vi "RGB to HSL.vi"(8 "Error In":errorcluster, 9 "Blue":u8, 10 "Green":u8, 11 "Red":u8) -> (0 "Error Out":errorcluster, 1 "Lum":u8, 2 "Sat":u8, 3 "Hue":u8)   [LabVIEW 2012, in "Picture Box Tools.lvlib"]
doc: "Converts RGB values (0-255) to HSL values (0-240). RGB colorspace is the display colorspace for web and computer monitors. RGB uses Red, Green and Blue components to form a color. This isn't very useful for programmatically changing a color. HSL colorspace uses Hue, Saturation and Lightness components of a color which can be analyzed, extract or modified in a way to change the function of a color. \n\nSee HSLToolsBasicExample.vi for more information in the NI Example Finder."
uses:
  Picture Box Tools.lvlib
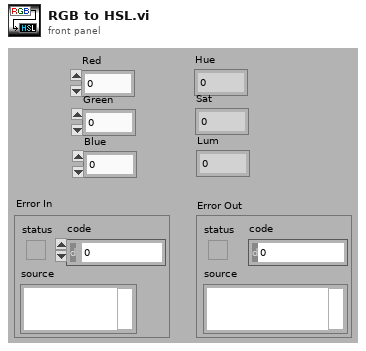
[diagram p1: front panel]
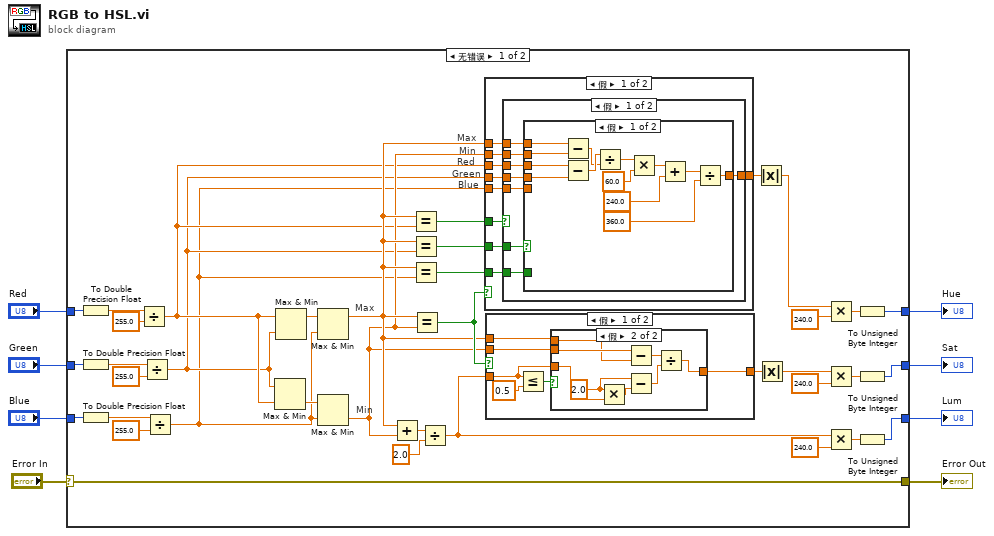
[diagram p0: block diagram]
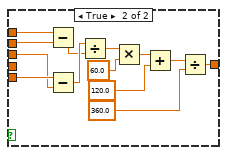
[diagram p2: hidden frame]
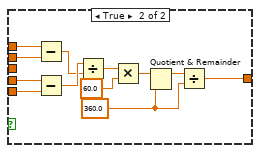
[diagram p3: hidden frame]
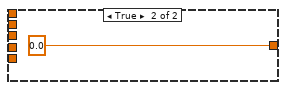
[diagram p4: hidden frame]
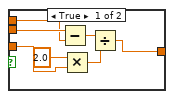
[diagram p5: hidden frame]
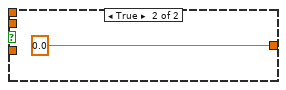
[diagram p6: hidden frame]
diagram:
  n1 = case shown="无错误" "Error In" {
    selector: "Error In" -> [w21 w124]
    tunnel: [w9 w127] -> w8
    tunnel: "Red" -> [w20 w127]
    tunnel: "Green" -> [w19 w126]
    tunnel: "Blue" -> [w18 w125]
    tunnel: [w10 w126] -> w4
    tunnel: [w11 w125] -> w3
    tunnel: [w21 w124] -> w1
    frame No Error {
      # "Blue"
      # "Green"
      # "Red"
      # "Min"
      # "Max"
      # "Min"
      # "Max"
      n2 = To Double Precision Float(number=w20) -> (double precision float=w17:dbl)
      n3 = To Double Precision Float(number=w19) -> (double precision float=w16:dbl)
      n4 = To Double Precision Float(number=w18) -> (double precision float=w15:dbl)
      n5 = Divide(x=w17, y=255.0) -> (x/y=w26:dbl)
      n6 = Divide(x=w16, y=255.0) -> (x/y=w25:dbl)
      n7 = Divide(x=w15, y=255.0) -> (x/y=w24:dbl)
      n8 = Max & Min(x=w25, y=w26) -> (min(x,y)=w44:dbl)  [unwired: 1 out]
      n9 = Max & Min(x=w26, y=w25) -> (max(x,y)=w45:dbl)  [unwired: 1 out]
      n10 = Max & Min(x=w45, y=w24) -> (max(x,y)=w28:dbl)  [unwired: 1 out]
      n11 = Max & Min(x=w44, y=w24) -> (min(x,y)=w27:dbl)  [unwired: 1 out]
      n12 = Add(x=w28, y=w27) -> (x+y=w42:dbl)
      n13 = Equal?(x=w28, y=w26) -> (x = y?=w29:bool)
      n14 = Equal?(x=w28, y=w25) -> (x = y?=w30:bool)
      n15 = Equal?(x=w28, y=w24) -> (x = y?=w31:bool)
      n16 = Equal?(x=w28, y=w27) -> (x = y?=w35:bool)
      n17 = Divide(x=w42, y=2.0) -> (x/y=w34:dbl)
      n18 = case shown="假" w35 {
        tunnel: w31 -> [w52 _]
        tunnel: w30 -> [w53 _]
        tunnel: w29 -> [w54 _]
        tunnel: w28 -> [w47 _]
        tunnel: w27 -> [w48 _]
        tunnel: w26 -> [w49 _]
        tunnel: w25 -> [w50 _]
        tunnel: w24 -> [w51 _]
        tunnel: [w46 0.0] -> w22
        frame False {
          n19 = case shown="假" w54 {
            tunnel: w53 -> [w62 _]
            tunnel: w52 -> [w61 _]
            tunnel: w51 -> [w60 w98]
            tunnel: w50 -> [w59 w99]
            tunnel: w49 -> [w58 _]
            tunnel: w48 -> [w57 w100]
            tunnel: w47 -> [w56 w97]
            tunnel: [w55 w89] -> w46
            frame False {
              n20 = case shown="假" w62 {
                tunnel: w61 -> [_ _]
                tunnel: w60 -> [_ w79]
                tunnel: w59 -> [w74 _]
                tunnel: w58 -> [w75 w78]
                tunnel: w57 -> [w72 w87]
                tunnel: w56 -> [w73 w88]
                tunnel: [w65 w80] -> w55
                frame False {
                  n21 = Subtract(x=w73, y=w72) -> (x-y=w63:dbl)
                  n22 = Subtract(x=w75, y=w74) -> (x-y=w64:dbl)
                  n23 = Divide(x=w64, y=w63) -> (x/y=w71:dbl)
                  n24 = Multiply(x=w71, y=60.0) -> (x*y=w69:dbl)
                  n25 = Add(x=w69, y=240.0) -> (x+y=w67:dbl)
                  n26 = Divide(x=w67, y=360.0) -> (x/y=w65:dbl)
                }
                frame True {
                  n27 = Subtract(x=w88, y=w87) -> (x-y=w76:dbl)
                  n28 = Subtract(x=w79, y=w78) -> (x-y=w77:dbl)
                  n29 = Divide(x=w77, y=w76) -> (x/y=w86:dbl)
                  n30 = Multiply(x=w86, y=60.0) -> (x*y=w84:dbl)
                  n31 = Add(x=w84, y=120.0) -> (x+y=w82:dbl)
                  n32 = Divide(x=w82, y=360.0) -> (x/y=w80:dbl)
                }
              }
            }
            frame True {
              w90 = 360.0 ("y")
              n33 = Subtract(x=w97, y=w100) -> (x-y=w95:dbl)
              n34 = Subtract(x=w99, y=w98) -> (x-y=w96:dbl)
              n35 = Divide(x=w96, y=w95) -> (x/y=w94:dbl)
              n36 = Multiply(x=w94, y=60.0) -> (x*y=w92:dbl)
              n37 = Quotient & Remainder(x=w92, y=w90) -> (x-y*floor(x/y)=w91:dbl)  [unwired: 1 out]
              n38 = Divide(x=w91, y=w90) -> (x/y=w89:dbl)
            }
          }
        }
        frame True {
        }
      }
      n39 = case shown="假" w35 {
        tunnel: [w102 0.0] -> w32
        tunnel: w34 -> [w103 _]
        tunnel: w27 -> [w105 _]
        tunnel: w28 -> [w104 _]
        frame False {
          n40 = Less Or Equal?(x=w103, y=0.5) -> (x <= y?=w106:bool)
          n41 = case shown="假" w106 {
            tunnel: w105 -> [w114 w122]
            tunnel: w104 -> [w113 w121]
            tunnel: w103 -> [w110 w119]
            tunnel: [w108 w118] -> w102
            frame True {
              n42 = Subtract(x=w114, y=w113) -> (x-y=w112:dbl)
              n43 = Multiply(x=2.0, y=w110) -> (x*y=w109:dbl)
              n44 = Divide(x=w112, y=w109) -> (x/y=w108:dbl)
            }
            frame False {
              w116 = 2.0 ("x")
              n45 = Multiply(x=w116, y=w119) -> (x*y=w117:dbl)
              n46 = Subtract(x=w122, y=w121) -> (x-y=w120:dbl)
              n47 = Subtract(x=w116, y=w117) -> (x-y=w115:dbl)
              n48 = Divide(x=w120, y=w115) -> (x/y=w118:dbl)
            }
          }
        }
        frame True {
        }
      }
      n49 = Absolute Value(x=w22) -> (abs(x)=w23:dbl)
      n50 = Absolute Value(x=w32) -> (abs(x)=w33:dbl)
      n51 = Multiply(x=w23, y=240.0) -> (x*y=w13:dbl)
      n52 = Multiply(x=w33, y=240.0) -> (x*y=w14:dbl)
      n53 = Multiply(x=w34, y=240.0) -> (x*y=w12:dbl)
      n54 = To Unsigned Byte Integer(number=w13) -> (unsigned 8bit integer=w9:u8)
      n55 = To Unsigned Byte Integer(number=w14) -> (unsigned 8bit integer=w10:u8)
      n56 = To Unsigned Byte Integer(number=w12) -> (unsigned 8bit integer=w11:u8)
    }
    frame Error {
    }
  }
  "Hue" <- w8
  "Sat" <- w4
  "Lum" <- w3
  "Error Out" <- w1
